vi "Parse Readings.vi"(11 "Readings":string) -> (2 "Measurement":T1 {"Measurement" format="%.6e"}, 3 "Remain Readings":string)   [LabVIEW 2016, in "Keithley 6517.lvlib"]
doc: "Parse the readings according to format."
uses:
  Keithley 6517.lvlib
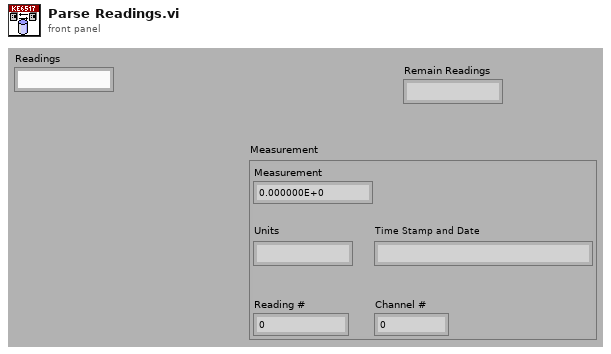
[diagram p1: front panel]
types:
  T1 = cluster{"Measurement":dbl, "Units":string, "Time Stamp and Date":string, "Reading #":dbl, "Channel #":dbl}
  T2 = cluster{dbl, "Readings":string, "Readings":string, dbl, dbl}
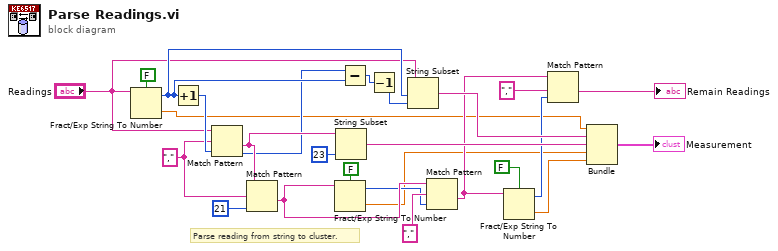
[diagram p0: block diagram]
diagram:
  w9 = ","
  # "Parse reading from string to cluster."
  n1 = Fract/Exp String To Number(use system decimal point (T)=FALSE, string="Readings") -> (offset past number=w19:i32, number=w4:dbl)  [unwired: 2 in]
  n2 = Increment(x=w19) -> (x+1=w18:i32)
  n3 = Match Pattern(string="Readings", regular expression=w9, offset (0)=w18) -> (after substring=w22:string, offset past match=w15:i32)  [unwired: 2 out]
  n4 = Match Pattern(string=w22, regular expression=w9, offset (0)=21) -> (after substring=w8:string)  [unwired: 3 out]
  n5 = Fract/Exp String To Number(use system decimal point (T)=FALSE, string=w8) -> (offset past number=w7:i32, number=w5:dbl)  [unwired: 2 in]
  n6 = String Subset(string=w22, length (rest)=23) -> (substring=w20:string)  [unwired: 1 in]
  n7 = Subtract(x=w15, y=w19) -> (x-y=w14:i32)
  n8 = Decrement(x=w14) -> (x-1=w17:i32)
  n9 = String Subset(string="Readings", offset (0)=w19, length (rest)=w17) -> (substring=w16:string)
  n10 = Match Pattern(string=w8, regular expression=",", offset (0)=w7) -> (after substring=w11:string)  [unwired: 3 out]
  n11 = Fract/Exp String To Number(use system decimal point (T)=FALSE, string=w11) -> (offset past number=w12:i32, number=w6:dbl)  [unwired: 2 in]
  n12 = Match Pattern(string=w11, regular expression=",", offset (0)=w12) -> (after substring=→"Remain Readings":string)  [unwired: 3 out]
  n13 = Bundle(w4, "Readings"=w16, "Readings"=w20, w5, w6) -> (→"Measurement":T2)  [unwired: 1 in]
